vi "Parse Binary String.vi"(8 "Error In":errorcluster, 10 "Tracker":T1, 11 "read buffer in":string) -> (0 "Error Out":errorcluster, 1 "Rigid Body Data":T2[](array[typedef]), 2 "Timestamp":dbl, 3 "Packet Data":T3)   [LabVIEW 2017]
uses:
  Controls/Packet Data.ctl
  Controls/Raw Rigid Body Data.ctl
  Controls/Tracker Type.ctl
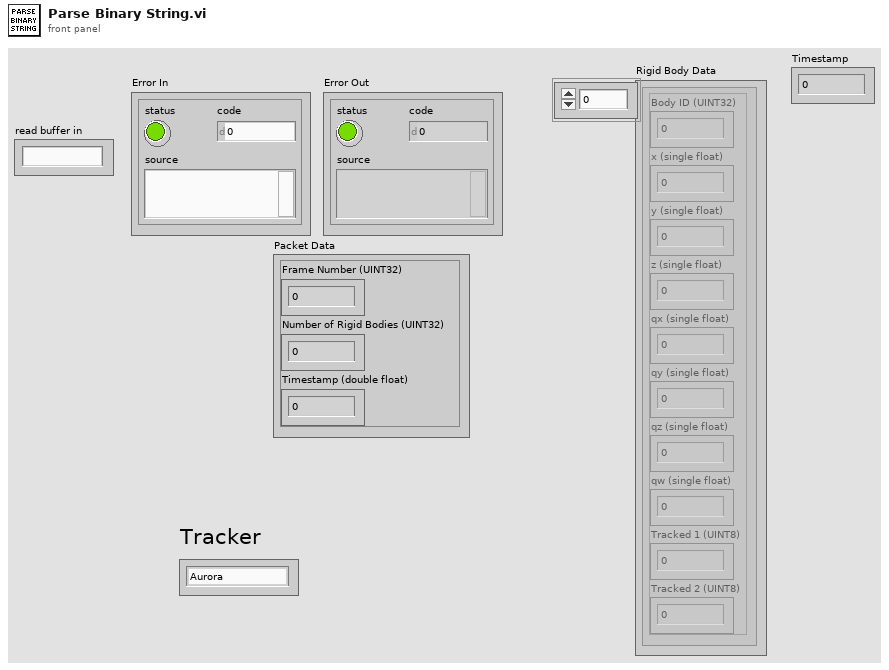
[diagram p1: front panel]
types:
  T1 = typedef "Tracker Type.ctl" = enum16{"Aurora", "OptiTrack"}
  T2 = typedef "Raw Rigid Body Data.ctl" = cluster{"Body ID (UINT32)":u32, "x (single float)":sgl, "y (single float)":sgl, "z (single float)":sgl, "qx (single float)":sgl, "qy (single float)":sgl, "qz (single float)":sgl, "qw (single float)":sgl, "Tracked 1 (UINT8)":u8, "Tracked 2 (UINT8)":u8}
  T3 = typedef "Packet Data.ctl" = cluster{"Frame Number (UINT32)":u32, "Number of Rigid Bodies (UINT32)":u32, "Timestamp (double float)":dbl}
  T4 = enum16{"big-endian, network order", "native, host order", "little-endian"}
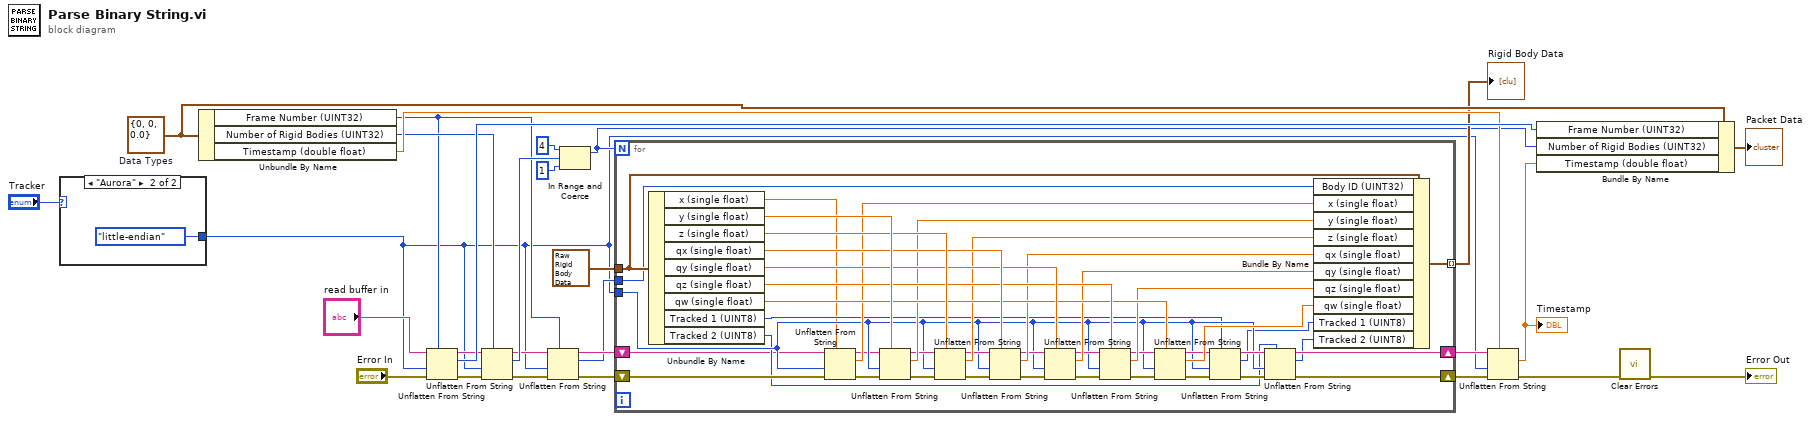
[diagram p0: block diagram]
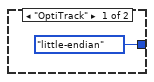
[diagram p2: hidden frame]
diagram:
  w28 = T3 {"Frame Number (UINT32)"=0, "Number of Rigid Bodies (UINT32)"=0, "Timestamp (double float)"=0.0}  # Data Types
  n1 = case shown="\"Aurora\"" "Tracker" {
    tunnel: [T4."little-endian" ("byte order (0:big-endian, network order)") T4."little-endian" ("byte order (0:big-endian, network order)")] -> w1
    frame "OptiTrack" {
    }
    frame "Aurora" {
    }
  }
  n2 = Unbundle By Name(w28) -> ("Frame Number (UINT32)"=w3:u32, "Number of Rigid Bodies (UINT32)"=w13:u32, "Timestamp (double float)"=w16:dbl)
  n3 = Unflatten From String(type=w3, binary string="read buffer in", byte order (0:big-endian, network order)=w1, error in (no error)="Error In") -> (rest of the binary string=w20:string, value=w27:u32, error out=w26:errorcluster)  [unwired: 1 in]
  n4 = Unflatten From String(type=w13, binary string=w20, byte order (0:big-endian, network order)=w1, error in (no error)=w26) -> (rest of the binary string=w5:string, value=w11:u32, error out=w7:errorcluster)  [unwired: 1 in]
  n5 = Unflatten From String(type=w3, binary string=w5, byte order (0:big-endian, network order)=w1, error in (no error)=w7) -> (rest of the binary string=w4:string, value=w2:u32, error out=w6:errorcluster)  [unwired: 1 in]
  n6 = In Range and Coerce(upper limit=u32 4, x=w11, lower limit=u32 1) -> (coerced(x)=w10:u32)  [unwired: 1 out]
  n7 = for {
    N: w10 -> [_]
    tunnel: [w72] -> w14 mode=indexing
    tunnel: T2 {"Body ID (UINT32)"=0, "x (single float)"=0.0, "y (single float)"=0.0, "z (single float)"=0.0, "qx (single float)"=0.0, "qy (single float)"=0.0, "qz (single float)"=0.0, "qw (single float)"=0.0, "Tracked 1 (UINT8)"=0, "Tracked 2 (UINT8)"=0} ("Rigid Body Data Types") -> [w35]
    shift-right: [w41] -> w18
    shift-left: w6 -> [w71]
    tunnel: w1 -> [w44]
    shift-right: [w40] -> w19
    shift-left: w4 -> [w34]
    tunnel: w2 -> [w31]
    n8 = Unbundle By Name(w35) -> ("x (single float)"=w32:sgl, "y (single float)"=w70:sgl, "z (single float)"=w69:sgl, "qx (single float)"=w63:sgl, "qy (single float)"=w62:sgl, "qz (single float)"=w61:sgl, "qw (single float)"=w60:sgl, "Tracked 1 (UINT8)"=w38:u8, "Tracked 2 (UINT8)"=w39:u8)
    n9 = Unflatten From String(type=w32, binary string=w34, byte order (0:big-endian, network order)=w44, error in (no error)=w71) -> (rest of the binary string=w33:string, value=w59:sgl, error out=w68:errorcluster)  [unwired: 1 in]
    n10 = Unflatten From String(type=w70, binary string=w33, byte order (0:big-endian, network order)=w44, error in (no error)=w68) -> (rest of the binary string=w52:string, value=w58:sgl, error out=w67:errorcluster)  [unwired: 1 in]
    n11 = Unflatten From String(type=w69, binary string=w52, byte order (0:big-endian, network order)=w44, error in (no error)=w67) -> (rest of the binary string=w51:string, value=w57:sgl, error out=w64:errorcluster)  [unwired: 1 in]
    n12 = Unflatten From String(type=w63, binary string=w51, byte order (0:big-endian, network order)=w44, error in (no error)=w64) -> (rest of the binary string=w50:string, value=w56:sgl, error out=w53:errorcluster)  [unwired: 1 in]
    n13 = Unflatten From String(type=w62, binary string=w50, byte order (0:big-endian, network order)=w44, error in (no error)=w53) -> (rest of the binary string=w49:string, value=w55:sgl, error out=w66:errorcluster)  [unwired: 1 in]
    n14 = Unflatten From String(type=w61, binary string=w49, byte order (0:big-endian, network order)=w44, error in (no error)=w66) -> (rest of the binary string=w48:string, value=w54:sgl, error out=w65:errorcluster)  [unwired: 1 in]
    n15 = Unflatten From String(type=w60, binary string=w48, byte order (0:big-endian, network order)=w44, error in (no error)=w65) -> (rest of the binary string=w46:string, value=w47:sgl, error out=w43:errorcluster)  [unwired: 1 in]
    n16 = Unflatten From String(type=w38, binary string=w46, byte order (0:big-endian, network order)=w44, error in (no error)=w43) -> (rest of the binary string=w45:string, value=w36:u8, error out=w42:errorcluster)  [unwired: 1 in]
    n17 = Unflatten From String(type=w39, binary string=w45, byte order (0:big-endian, network order)=w44, error in (no error)=w42) -> (rest of the binary string=w40:string, value=w37:u8, error out=w41:errorcluster)  [unwired: 1 in]
    n18 = Bundle By Name(cluster=w35, "Body ID (UINT32)"=w31, "x (single float)"=w59, "y (single float)"=w58, "z (single float)"=w57, "qx (single float)"=w56, "qy (single float)"=w55, "qz (single float)"=w54, "qw (single float)"=w47, "Tracked 1 (UINT8)"=w36, "Tracked 2 (UINT8)"=w37) -> (w72:T2)
  }
  "Rigid Body Data" <- w14
  n19 = Unflatten From String(type=w16, binary string=w19, byte order (0:big-endian, network order)=w1, error in (no error)=w18) -> (value=w15:dbl, error out=w17:errorcluster)  [unwired: 1 in, 1 out]
  "Timestamp" <- w15
  n20 = Bundle By Name(cluster=w28, "Frame Number (UINT32)"=w27, "Number of Rigid Bodies (UINT32)"=w10, "Timestamp (double float)"=w15) -> (→"Packet Data":T3)
  n21 = call <vilib>:"Clear Errors.vi"("error in (no error)"=w17) -> ("error out"=→"Error Out":errorcluster)  [unwired: 5 in, 1 out]
